vi "Reset Manipulator Controls.vi"(11 "Operator Buttons":bool[](array[boolean])) -> (2 "Reset Requested?":bool, 3 "Reset Parameters":T1)   [LabVIEW 2020]
uses:
  <vilib>/Rock Robotics/WPI/Joystick/XBox Buttons Indexer.ctl
  f6c53150-5c8e-4723-8b9f-f8d1b2b2ef89.vi
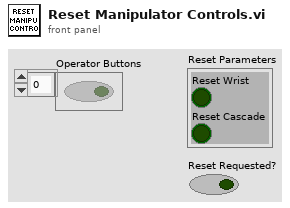
[diagram p1: front panel]
types:
  T1 = cluster{"Reset Wrist":bool, "Reset Cascade":bool}
  T2 = typedef "XBox Buttons Indexer.ctl" = enum16{"A", "B", "X", "Y", "Left Bumper", "Right Bumper", "Back", "Start", "Left Joystick", "Right Joystick"}
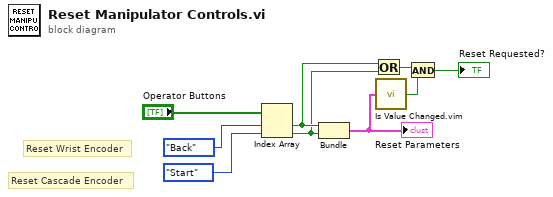
[diagram p0: block diagram]
diagram:
  # "Reset Cascade Encoder"
  # "Reset Wrist Encoder"
  n1 = Index Array(array="Operator Buttons", index #1=XBox_Buttons_Indexer."Back" ("XBox Buttons"), index #2=XBox_Buttons_Indexer."Start" ("XBox Buttons")) -> (element #1=w6:bool, element #2=w5:bool)
  n2 = Bundle(w6, w5) -> (w4:cluster{bool, bool})  [unwired: 1 in]
  "Reset Parameters" <- w4
  n3 = Or(x=w6, y=w5) -> (x .or. y?=w3:bool)
  n4 = call "Is Value Changed.vim"("value"=w4) -> ("changed or first call?"=w2:bool)
  n5 = And(x=w3, y=w2) -> (x .and. y?=→"Reset Requested?":bool)
